vi "start.vi"(8 "error in (no error)":errorcluster, 11 "DAQmx_pulse_out in":refnum<class "DAQmx_pulse_out.lvclass">) -> (0 "error out":errorcluster, 3 "DAQmx_pulse_out out":refnum<class "DAQmx_pulse_out.lvclass">)   [LabVIEW 2013, in "DAQmx_pulse_out.lvclass"]
uses:
  DAQmx_pulse_out.lvclass
  DAQmx_pulse_out.lvclass/DAQmx_pulse_out.ctl
  Experiment/Globals.vi
  Experiment/Experiment.lvclass
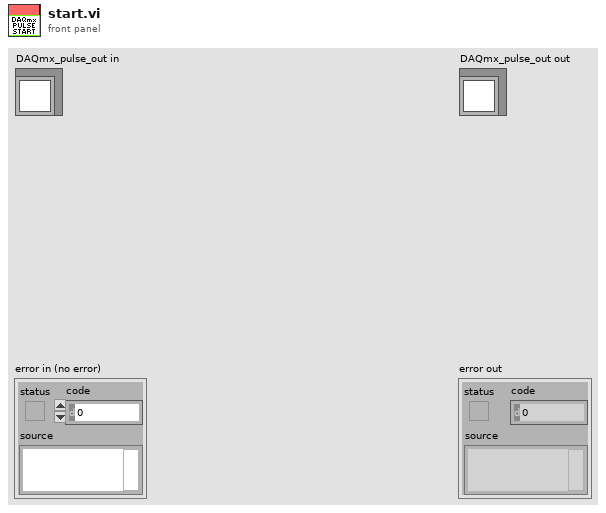
[diagram p1: front panel]
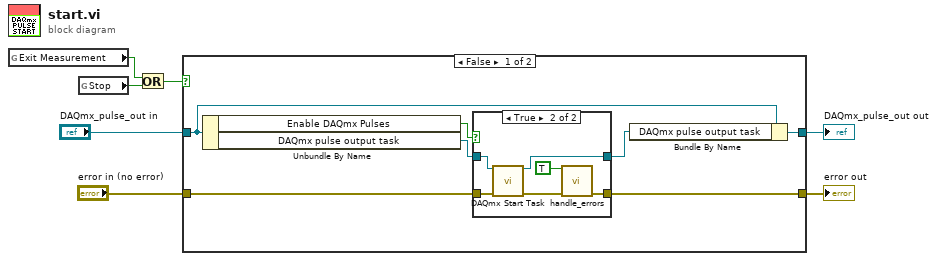
[diagram p0: block diagram]
diagram:
  n1 = global read "Globals.vi" "Exit Measurement"() -> (w3:bool)
  n2 = global read "Globals.vi" "Stop"() -> (w4:bool)
  n3 = Or(x=w3, y=w4) -> (x .or. y?=w2:bool)
  n4 = case shown="False" w2 {
    tunnel: [w9 w23] -> w7
    tunnel: [w11 w24] -> w5
    tunnel: "DAQmx_pulse_out in" -> [w12 w24]
    tunnel: "error in (no error)" -> [w8 w23]
    frame False {
      n5 = Unbundle By Name(w12) -> ("Enable DAQmx Pulses"=w14:bool, "DAQmx pulse output task"=w13:refnum<k21>)
      n6 = case shown="True" w14 {
        tunnel: w8 -> [w16 w22]
        tunnel: w13 -> [w15 w21]
        tunnel: [w16 w17] -> w9
        tunnel: [w15 w20] -> w10
        frame False {
        }
        frame True {
          n7 = call <vilib>:"DAQmx Start Task.vi"("task/channels in"=w21, "error in"=w22) -> ("task out"=w20:refnum<k21>, "error out"=w18:errorcluster)  [unwired: 12 in]
          n8 = call "handle_errors.vi"("Exit Operation"=TRUE ("Exit Measurement"), "error in (no error)"=w18) -> ("error out"=w17:errorcluster)  [unwired: 13 in]
        }
      }
      n9 = Bundle By Name(cluster=w12, "DAQmx pulse output task"=w10) -> (w11:refnum<class "DAQmx_pulse_out.lvclass">)
    }
    frame True {
    }
  }
  "error out" <- w7
  "DAQmx_pulse_out out" <- w5
